vi "Enable Heartbeat.vi"(8 "error in":errorcluster, 9 "Period":u32 format="%d ms", 10 "Node ID":u8, 11 "CANopen Actor Interface in":refnum<class "CANopen Actor Interface.lvclass">) -> (0 "error out":errorcluster, 3 "CANopen Actor Interface out":refnum<class "CANopen Actor Interface.lvclass">)   [LabVIEW 2024, in "CANopen Actor Interface.lvlib" / "CANopen Actor Interface.lvclass"]
uses:
  CANopen Actor Interface.lvclass
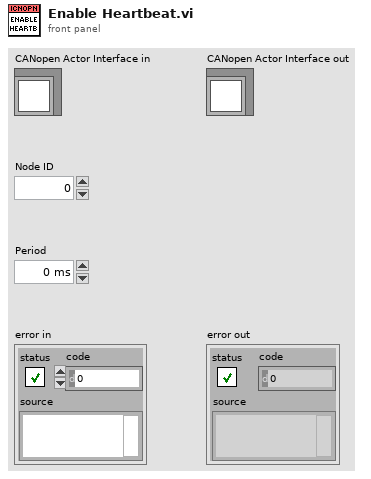
[diagram p1: front panel]
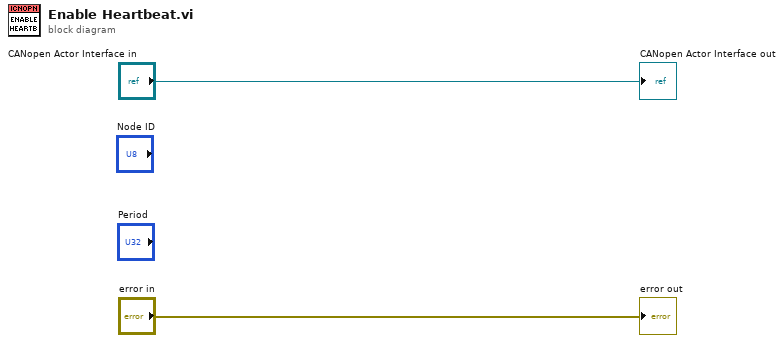
[diagram p0: block diagram]
diagram:
  "error out" <- "error in"
  "CANopen Actor Interface out" <- "CANopen Actor Interface in"
